vi "Get Active Worksheet.vi"(8 "error in (no error)":errorcluster, 11 "Excel Interface in":refnum<class "Excel Interface.lvclass">) -> (0 "error out":errorcluster, 2 "Excel Sheet out":refnum<class "Excel Sheet.lvclass">, 3 "Excel Interface out":refnum<class "Excel Interface.lvclass">)   [LabVIEW 2016, in "Excel Interface.lvclass"]
uses:
  Excel Interface.lvclass
  Excel Sheet/Excel Sheet.lvclass
  Excel Interface.lvclass/Excel Interface.ctl
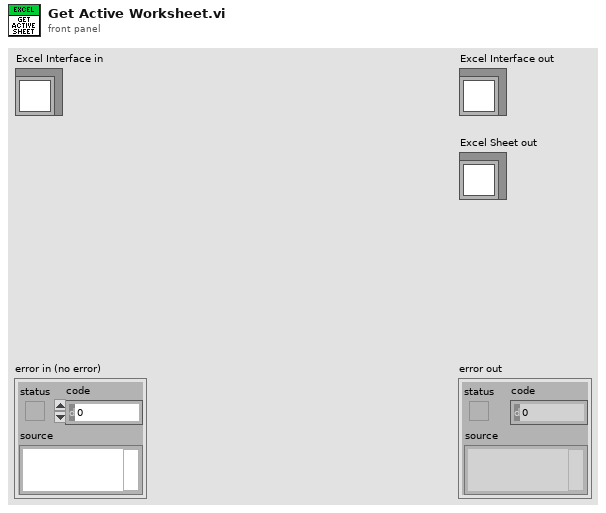
[diagram p1: front panel]
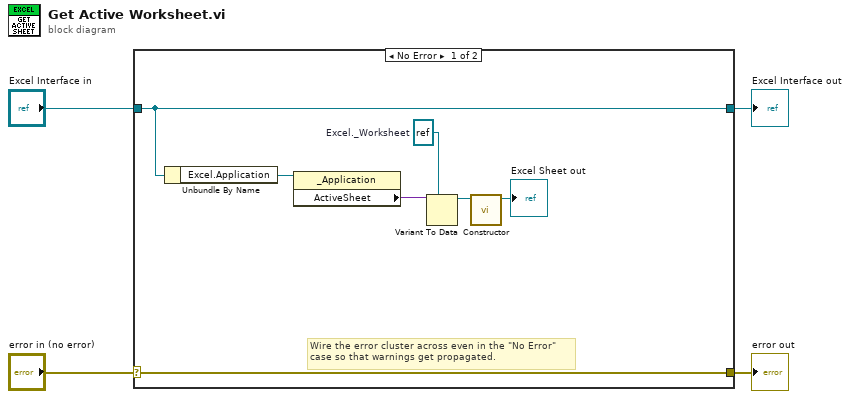
[diagram p0: block diagram]
diagram:
  n1 = case shown="No Error" "error in (no error)" {
    selector: "error in (no error)" -> [w11 w13]
    tunnel: [w11 w13] -> w3
    tunnel: [w10 w12] -> w1
    tunnel: "Excel Interface in" -> [w10 w12]
    frame No Error {
      w7 = refnum<k7> refnum  # Excel._Worksheet
      # "Wire the error cluster across even in the \"No Error\"\ncase so that warnings get propagated."
      n2 = Unbundle By Name(w10) -> ("Excel.Application"=w9:refnum<k7>)
      n3 = property class="_Application"(reference=w9) -> ("ActiveSheet"=w8:variant)  [unwired: 1 in, 2 out]
      n4 = Variant To Data(type=w7, Variant=w8) -> (data=w6:refnum<k7>)  [unwired: 1 in, 1 out]
      n5 = call "Constructor.vi"("Worksheet"=w6) -> ("Excel Sheet out"=→"Excel Sheet out":refnum<class "Excel Sheet.lvclass">)  [unwired: 10 in]
    }
    frame Error {
    }
  }
  "error out" <- w3
  "Excel Interface out" <- w1
